vi "readTag.vi"(8 "error in (no error)":errorcluster, 11 "OPC in":refnum<class "OPC.lvclass">) -> (0 "error out":errorcluster, 3 "OPC out":refnum<class "OPC.lvclass">)   [LabVIEW 2020, in "OPC.lvclass"]
uses:
  OPC.lvclass
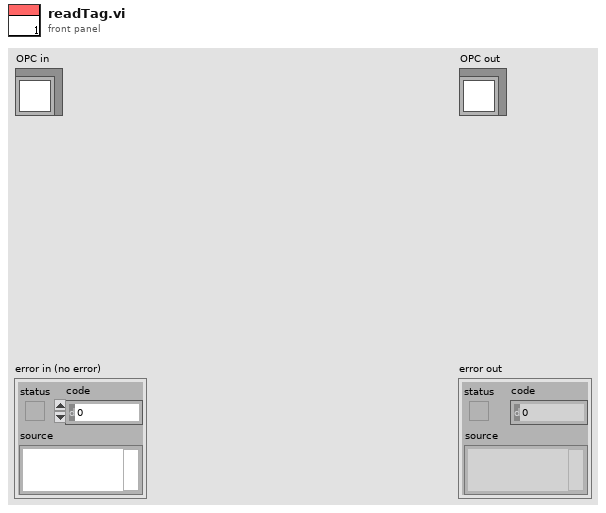
[diagram p1: front panel]
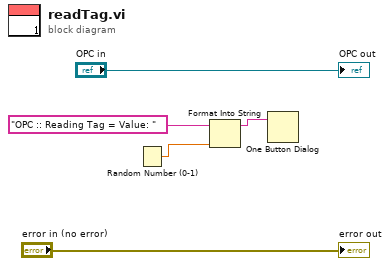
[diagram p0: block diagram]
diagram:
  n1 = Random Number (0-1)() -> (number: 0 to 1=w2:dbl)
  n2 = Format Into String(initial string="OPC :: Reading Tag = Value: " ("message"), w2) -> (resulting string=w1:string)  [unwired: 2 in, 1 out]
  n3 = One Button Dialog(message=w1) -> ()  [unwired: 1 in, 1 out]
  "error out" <- "error in (no error)"
  "OPC out" <- "OPC in"
